vi "get-signal-payload.vi"(7 "frame.tag":string, 8 "error in (no error)":errorcluster, 9 "bit.len":i32, 10 "start.pos":i32, 11 "CANtable in":refnum<class "bAPPdata.lvclass">) -> (0 "error out":errorcluster, 2 "payload":u32, 3 "CANtable out":refnum<class "bAPPdata.lvclass">)   [LabVIEW 2015, in "bAPPdata.lvclass"]
uses:
  bAPPdata.lvclass
  bAPPdata.lvclass/bAPPdata.ctl
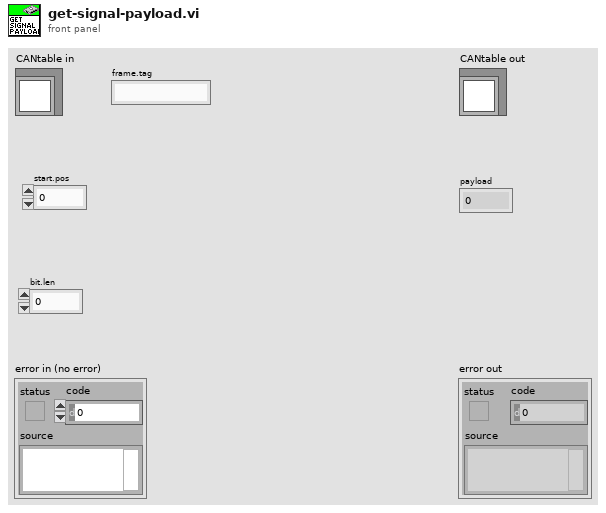
[diagram p1: front panel]
types:
  T1 = typedef "bAPPdata.lvclass/table-data.ctl" = T2[]
  T2 = typedef "bAPPdata.lvclass/table-contents.ctl" = cluster{"id":u32, "tag":string, "frame.type":T3, "last.frame":T4, "tMsgData":T6, "child.tags":string[], "bit-payload":bool[]}
  T3 = typedef "frame.type.ctl" = enum16{"FRAME NOT DEFINED", "DUT OUTPUT FRAME", "DUT INPUT FRAME"}
  T4 = typedef "XNET Frame CAN.ctl" = cluster{"timestamp":timestamp, "payload":u8[], "identifier":u32, "type":T5, "extended?":bool, "echo?":bool}
  T5 = typedef "XNET Frame Type CAN.ctl" = u8
  T6 = typedef "nMsgData.ctl" = cluster{"dwID":u32, "count":u32, "dwCycleTime":dbl, "dwTime":dbl, "new msg":bool}
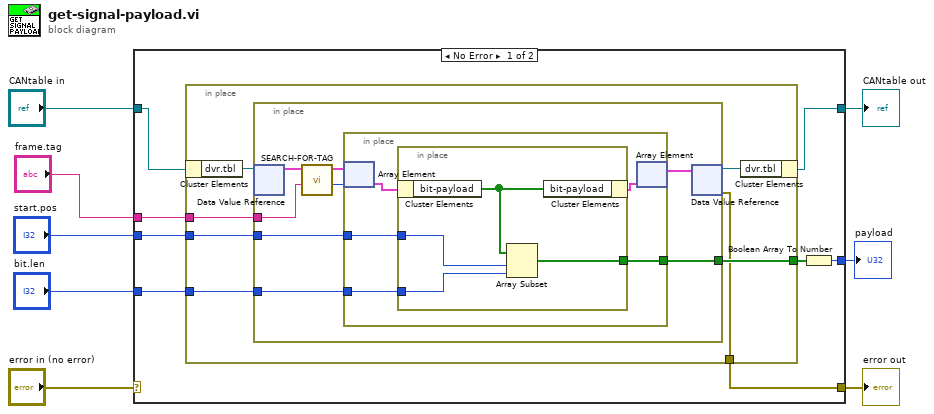
[diagram p0: block diagram]
diagram:
  n1 = case shown="No Error" "error in (no error)" {
    selector: "error in (no error)" -> [_ w42]
    tunnel: [w10 w42] -> w7
    tunnel: [w15 w41] -> w5
    tunnel: "CANtable in" -> [w16 w41]
    tunnel: [w9 _] -> w1
    tunnel: "bit.len" -> [w13 _]
    tunnel: "start.pos" -> [w12 _]
    tunnel: "frame.tag" -> [w11 _]
    frame No Error {
      n2 = in-place {
        in-place-border: [w21] -> w14
        in-place-border: w13 -> [w20]
        in-place-border: w12 -> [w19]
        in-place-border: w11 -> [w18]
        in-place-border: [w17] -> w10
        n3 = in-place-cluster #1(w16) -> ("dvr.tbl"=w23:refnum<data-value>)
        n4 = in-place {
          in-place-border: [w29] -> w21
          in-place-border: w20 -> [w28]
          in-place-border: w19 -> [w27]
          in-place-border: w18 -> [w24]
          n5 = in-place-dvr #2(w23) -> (w31:T1)  [unwired: 1 out]
          n6 = call "SEARCH-FOR-TAG.vi"("tag"=w24, "tbl.list"=w31) -> ("idx"=w25:i32, "tbl.list out"=w26:T2[])  [unwired: 8 in]
          n7 = in-place {
            in-place-border: [w34] -> w29
            in-place-border: w28 -> [w33]
            in-place-border: w27 -> [w32]
            n8 = in-place-array #3(w26, w25) -> (w36:T2)
            n9 = in-place {
              in-place-border: [w39] -> w34
              in-place-border: w33 -> [w38]
              in-place-border: w32 -> [w37]
              n10 = in-place-cluster #4(w36) -> ("bit-payload"=w40:bool[])
              n11 = Array Subset(array=w40, index=w37, length=w38) -> (w39:bool[])
              n12 = in-place-cluster #4("bit-payload"=w40) -> (w35:T2)
            }
            n13 = in-place-array #3(w35) -> (w30:T2[])  [unwired: 1 out]
          }
          n14 = in-place-dvr #2(w30) -> (w22:refnum<data-value>, w17:errorcluster)
        }
        n15 = in-place-cluster #1("dvr.tbl"=w22) -> (w15:refnum<class "bAPPdata.lvclass">)
      }
      n16 = Boolean Array To Number(Boolean array=w14) -> (number=w9:u32)
    }
    frame Error {
    }
  }
  "error out" <- w7
  "CANtable out" <- w5
  "payload" <- w1
